vi "Live Report.vi"(8 "error in":errorcluster, 11 "TDMS in":refnum<class "TDMS.lvclass">) -> (0 "error out":errorcluster, 3 "TDMS out":refnum<class "TDMS.lvclass">)   [LabVIEW 2019, in "TDMS.lvlib" / "TDMS.lvclass"]
uses:
  TDMS.lvclass
  TDMS.lvclass/TDMS.ctl
  Report Viewer/Custom Controls/Browse Tools.ctl
  <vilib>/Utility/tdmsutil.llb/fileViewerConfigData.ctl
  Report Viewer/Report Viewer.lvclass
panel:
  out "TDMS File":string="Press 'Refresh Data' to load the latest data from the live report."
  in  "Display Format":T1(ring)
  in  "Refresh Data":bool
  in  "Save Data":bool
  in  "Settings":bool
  in  "Save Graph":bool
  in  "Finished":bool
  in  "File contents":string[](tree)=["\"\u0000\u0000\u0000\u0002\u0000\u0000\u0000+Halt Mode Running_11:25:18.755 AM 11/6/2019\u0000\u0000\u0000\nPJB1_S CH0\""]
  in  "Properties / Values / Graph":T2(tab)=enum."Analog values (graph)"
  in  "Properties":i32(listbox)
  in  "Raw data values":i32(listbox)=-1
  out "Waveform Graph":waveform(dbl)[](graph)=[{"t0"=timestamp(0 s since 1904-01-01), "dt"=1.0, "Y"=[]}]
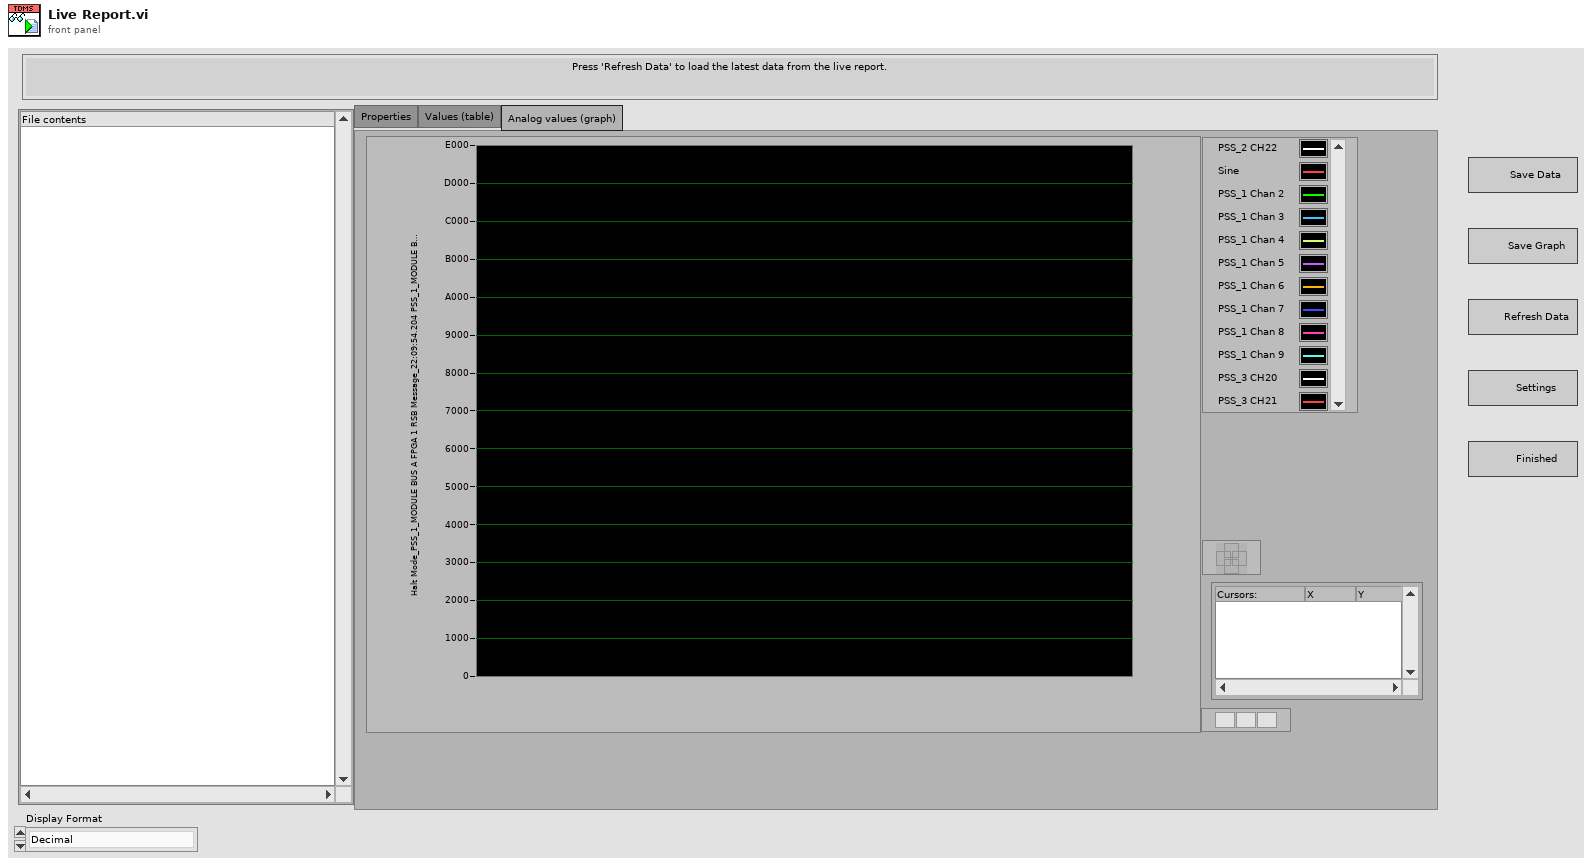
[diagram p1: front panel]
types:
  T1 = enum16{"Decimal", "Scientific", "Engineering", "Binary", "Octal", "Hexadecimal"}
  T2 = enum32{"Properties", "Values (table)", "Analog values (graph)"}
  T3 = typedef "fileViewerConfigData.ctl" = cluster{"Show all (table)":bool, "Show all (graph)":bool, "limit (table)":u64, "limit (graph)":u64, "no show":bool, "start (table)":u64, "start (graph)":u64}
  T4 = typedef "Report Viewer.lvlib/Report Viewer.lvclass/Browse Tools.ctl" = cluster{"Group":string, "Channel":string, "TDMS View Cfg":T3}
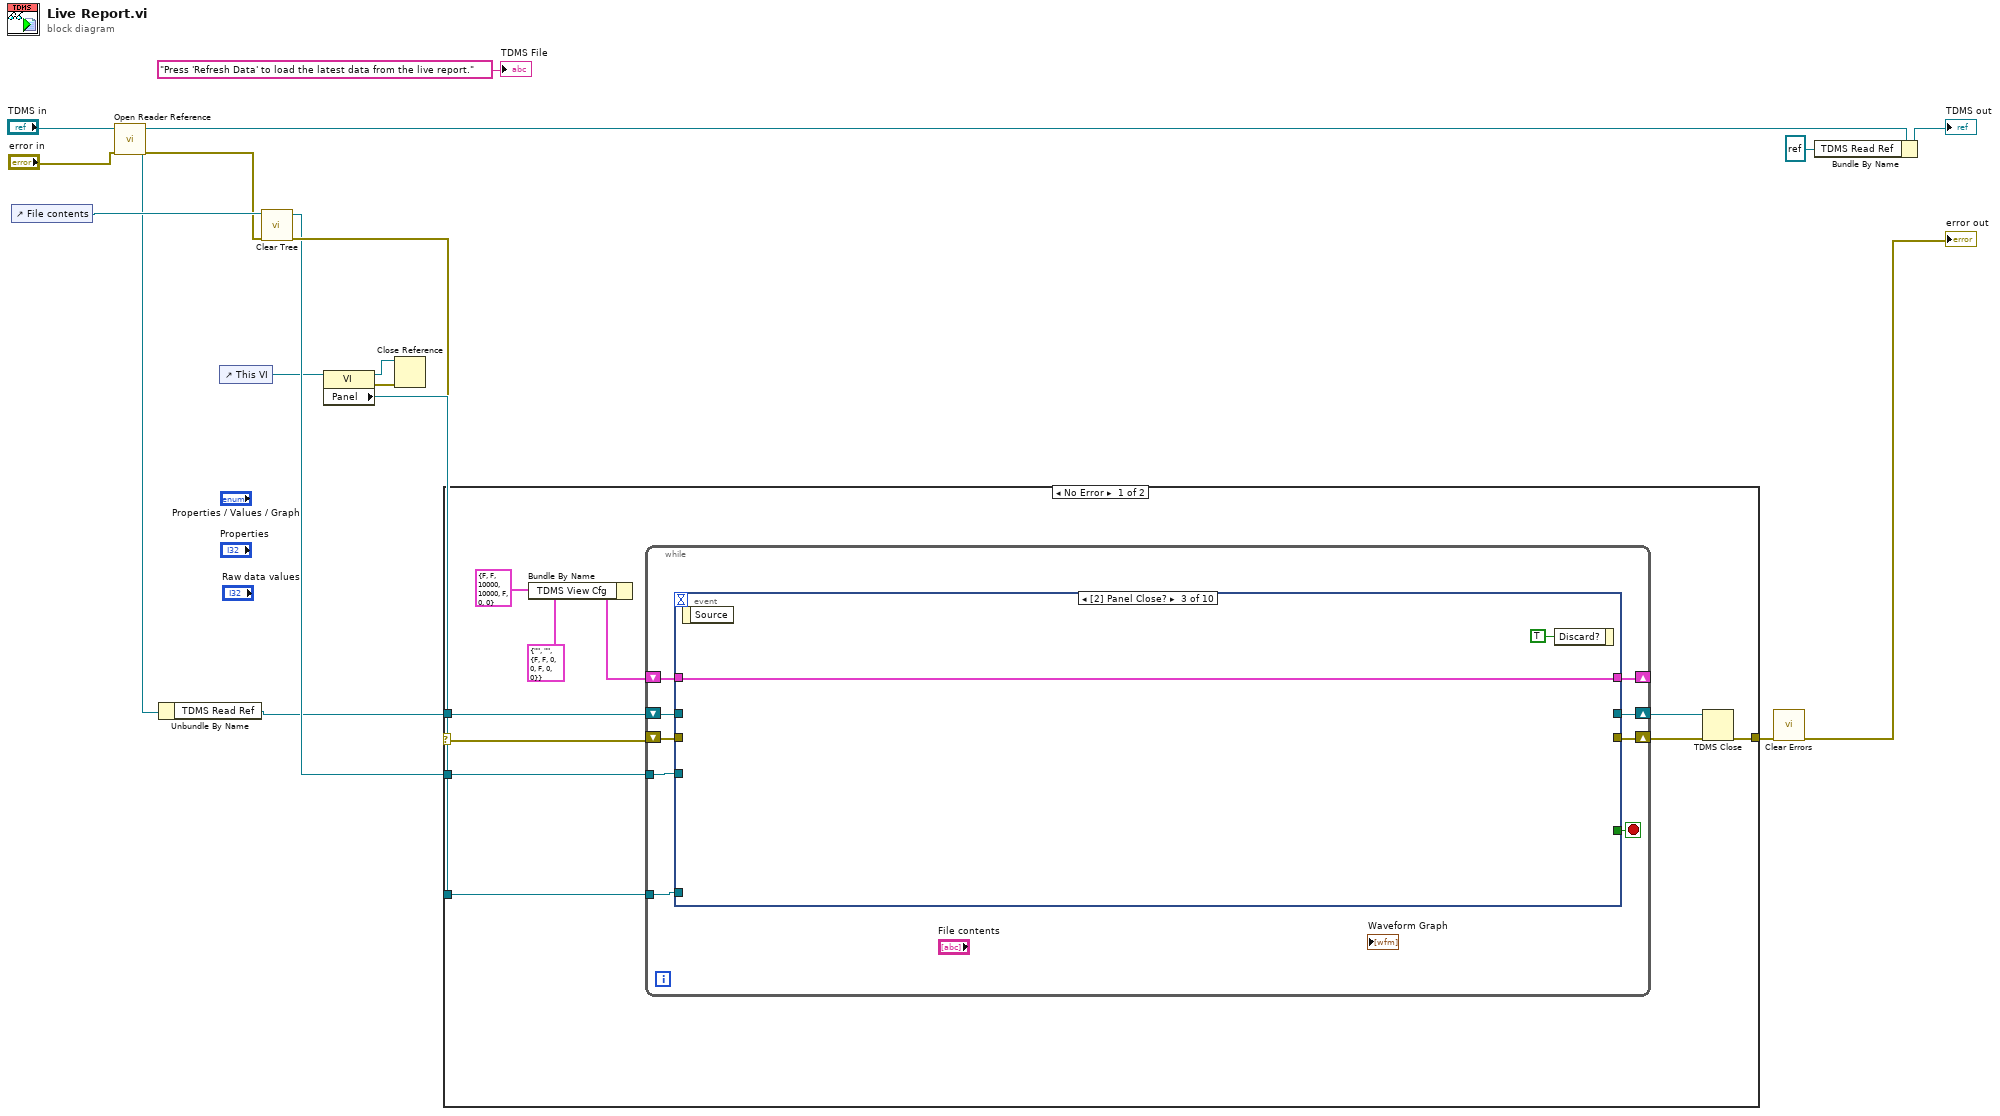
[diagram p0: block diagram]
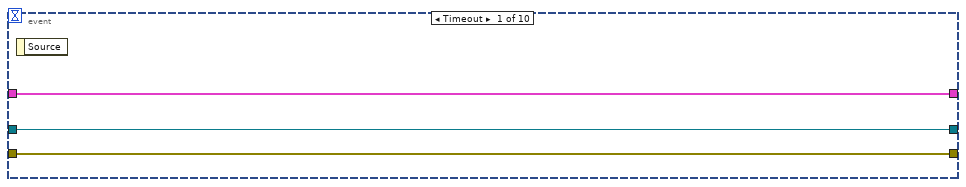
[diagram p2: hidden frame]
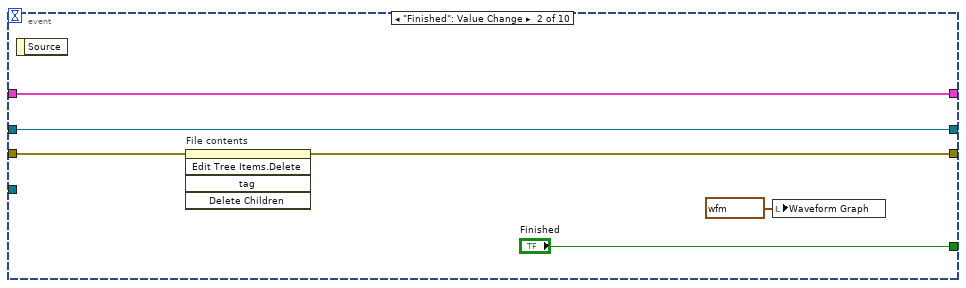
[diagram p3: hidden frame]
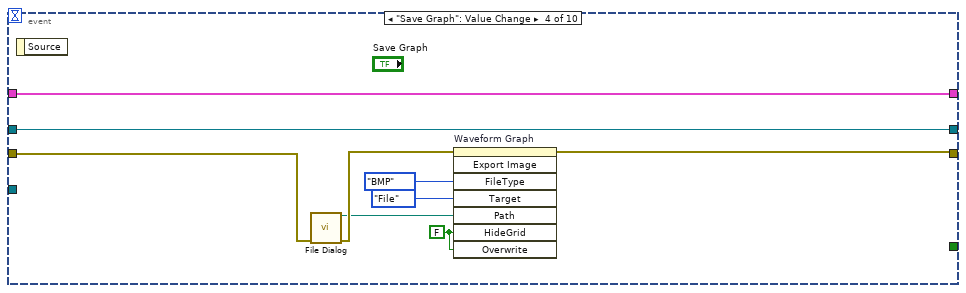
[diagram p4: hidden frame]
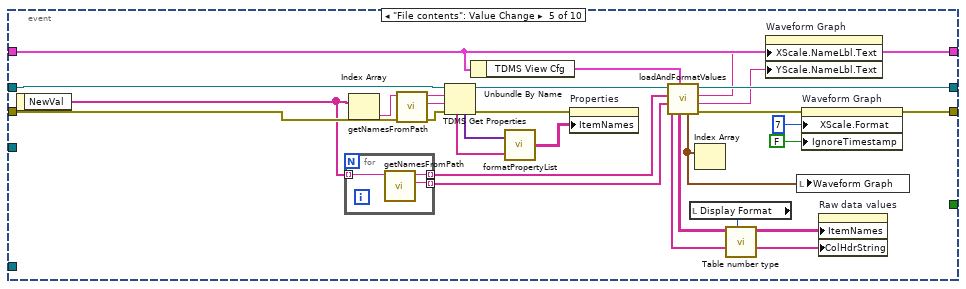
[diagram p5: hidden frame]
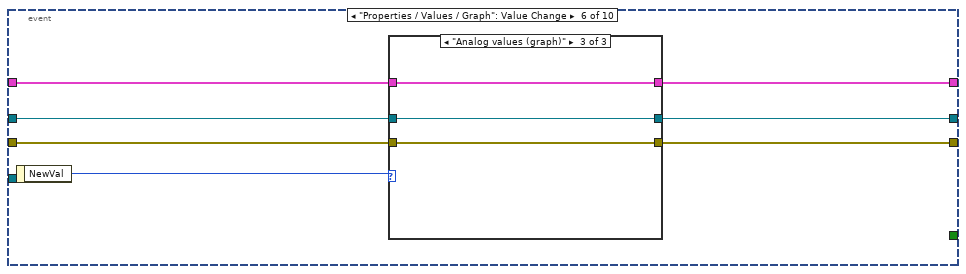
[diagram p6: hidden frame]
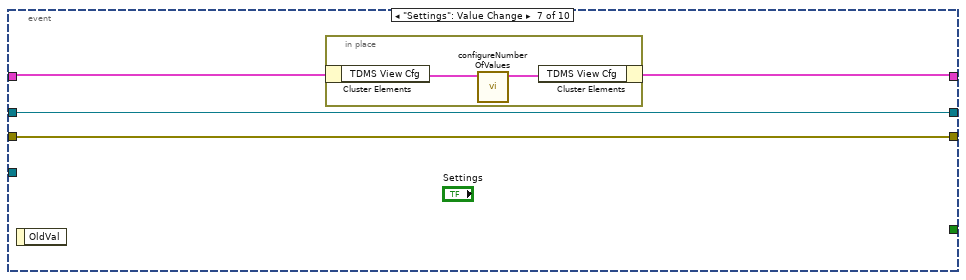
[diagram p9: hidden frame]
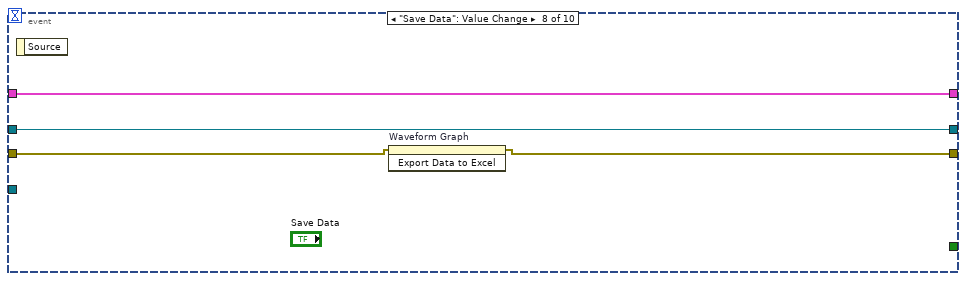
[diagram p10: hidden frame]
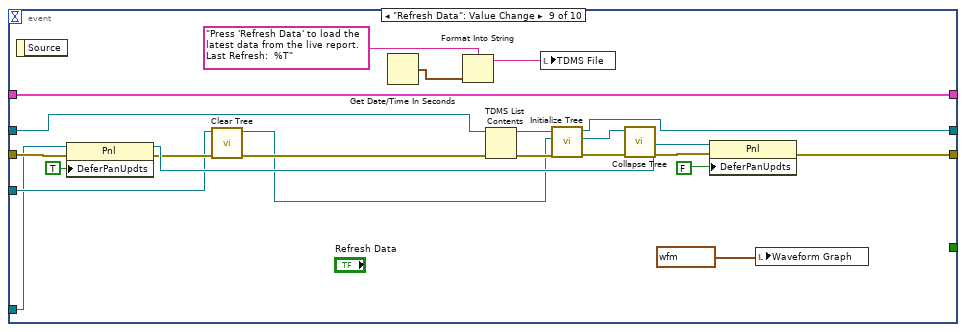
[diagram p11: hidden frame]
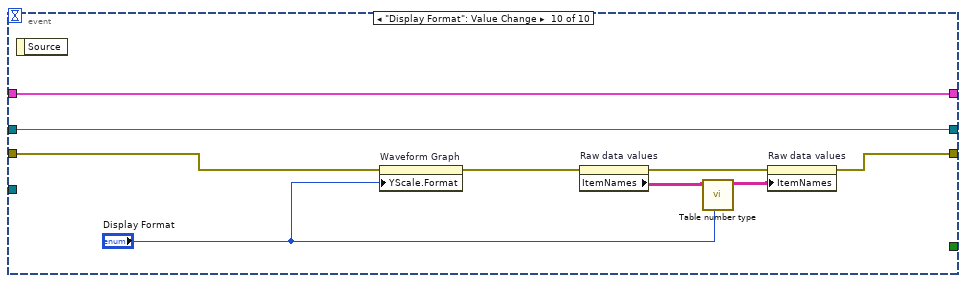
[diagram p12: hidden frame]
diagram:
  n1 = control-ref of="File contents"() -> (w16:refnum<vi>)
  n2 = call "Open Reader Reference.vi"("error in"="error in", "TDMS in"="TDMS in") -> ("error out"=w5:errorcluster, "TDMS out"=w4:refnum<class "TDMS.lvclass">)  [unwired: 8 in]
  n3 = Unbundle By Name(w4) -> ("TDMS Read Ref"=w6:refnum<k34>)
  n4 = control-ref of="This VI"() -> (w10:refnum<vi>)
  n5 = call "Clear Tree.vi"("error in"=w5, "reference"=w16) -> ("error out"=w14:errorcluster, "reference out"=w13:refnum<vi>)  [unwired: 8 in]
  n6 = property class="VI"(reference=w10) -> (reference out=w12:refnum<vi>, error out=w11:errorcluster, "Panel"=w15:refnum<vi>)  [unwired: 1 in]
  n7 = Close Reference(reference=w12, error in (no error)=w11) -> ()  [unwired: 1 out]
  n8 = case shown="No Error" w14 {
    selector: w14 -> [w20 w144]
    tunnel: [w27 w144] -> w9
    tunnel: w13 -> [w22 _]
    tunnel: w15 -> [w19 _]
    tunnel: w6 -> [w18 _]
    frame No Error {
      n9 = Bundle By Name(cluster=T4 {"Group"="", "Channel"="", "TDMS View Cfg"={"Show all (table)"=FALSE, "Show all (graph)"=FALSE, "limit (table)"=0, "limit (graph)"=0, "no show"=FALSE, "start (table)"=0, "start (graph)"=0}} ("Cluster"), "TDMS View Cfg"=T3 {"Show all (table)"=FALSE, "Show all (graph)"=FALSE, "limit (table)"=10000, "limit (graph)"=10000, "no show"=FALSE, "start (table)"=0, "start (graph)"=0} ("TDMS File Viewer Configuration")) -> (w24:T4)
      n10 = while {
        shift-right: [w34] -> w26
        shift-left: w20 -> [w35]
        shift-right: [w29] -> w21
        shift-left: w18 -> [w36]
        shift-right: [w31] -> _
        shift-left: w24 -> [w32]
        tunnel: w22 -> [w30]
        tunnel: w19 -> [w28]
        stop <- w33 stop-if-true
        n11 = event shown="[2] Panel Close?" {
          selector: _ -> [_ _ _ _ _ _ _ _ _ _]
          dyn-events: _ -> [_ _ _ _ _ _ _ _ _ _]
          timeout: _ -> [_ _ _ _ _ _ _ _ _ _]
          tunnel: w36 -> [w37 w42 _ w47 w61 w92 w103 w109 w118 w141]
          tunnel: w35 -> [w39 w40 _ w54 w83 w88 w104 w111 w124 w142]
          tunnel: [w39 w40 _ w53 w66 w87 w104 w110 w128 w139] -> w34
          tunnel: [_ "Finished" _ _ _ _ _ _ _ _] -> w33
          tunnel: w32 -> [w38 w43 w46 w55 w74 w91 w106 w112 w134 w143]
          tunnel: [w38 w43 w46 w55 w74 w90 w105 w112 w134 w143] -> w31
          tunnel: w30 -> [_ _ _ _ _ _ _ _ w121 _]
          tunnel: [w37 w42 _ w47 w62 w89 w103 w109 w127 w141] -> w29
          tunnel: w28 -> [_ _ _ _ _ _ _ _ w120 _]
          event Timeout {
            n12 = event-data() -> ()  [unwired: 1 in, 1 out]
          }
          event "Finished": Value Change {
            n13 = event-data() -> ()  [unwired: 1 in, 1 out]
            n14 = invoke on="File contents" class="Tree (strict)" method="Edit Tree Items.Delete"(error in=w40) -> ()  [unwired: 4 in, 5 out]
            n15 = local write "Waveform Graph"(waveform(dbl)[] [{"t0"=timestamp(0 s since 1904-01-01), "dt"=1.0, "Y"=[]}] ("Waveform Graph")) -> ()
          }
          event Panel Close? {
            n16 = event-data() -> ()  [unwired: 1 in, 1 out]
            n17 = event-data("Discard?"=TRUE) -> ()  [unwired: 1 in, 1 out]
          }
          event "Save Graph": Value Change {
            w48 = FALSE ("Hide Grid")
            n18 = event-data() -> ()  [unwired: 1 in, 1 out]
            n19 = call "File Dialog"("error in"=w54) -> ("selected path"=w49:path, "error out"=w52:errorcluster)  [unwired: 11 in, 2 out]
            n20 = invoke on="Waveform Graph" class="WFGraph (strict)" method="Export Image"(error in=w52, "FileType"=enum32{"BMP", "EPS", "EMF", "PICT"}."BMP" ("File Type"), "Target"=enum32{"File", "Clipboard"}."File", "Path"=w49, "HideGrid"=w48, "Overwrite"=w48) -> (error out=w53:errorcluster)  [unwired: 2 in, 7 out]
          }
          event "File contents": Value Change {
            n21 = event-data() -> ("NewVal"=w71:string[])  [unwired: 1 in]
            n22 = for {
              tunnel: w71 -> [w86] mode=indexing
              tunnel: [w85] -> w70 mode=indexing
              tunnel: [w84] -> w69 mode=indexing
              n23 = call <vilib>:"getNamesFromPath.vi"("tree path"=w86) -> ("channel"=w84:string, "group"=w85:string)  [unwired: 1 in, 4 out]
            }
            n24 = Index Array(array=w71) -> (element=w75:string)  [unwired: 1 in]
            n25 = call <vilib>:"getNamesFromPath.vi"("error in (no error)"=w83, "tree path"=w75) -> ("error out"=w82:errorcluster, "channel"=w80:string, "group"=w81:string)  [unwired: 3 out]
            n26 = TDMS Get Properties(8:w82, 9:w80, 10:w81, 11:w61) -> (0:w76:errorcluster, 3:w72:refnum<k34>, 4:w79:variant[], 6:w78:string[])  [unwired: 4 out]
            n27 = Unbundle By Name(w74) -> ("TDMS View Cfg"=w73:T3)
            n28 = call <vilib>:"formatPropertyList.vi"("property names"=w78, "property values"=w79) -> ("strings"=w77:string[][])
            n29 = property on="Properties" class="MCListbox (strict)"(error in=w76, "ItemNames"=w77) -> ()  [unwired: 1 in, 2 out]
            n30 = call <vilib>:"loadAndFormatValues.vi"("configuration"=w73, "channel names"=w69, "group names"=w70, "tdms file"=w72) -> ("error out"=w67:errorcluster, "graph y names"=w59:string, "graph x names"=w60:string, "tdms file out"=w62:refnum<k34>, "waveform values"=w63:waveform(dbl)[], "table values"=w57:string[][], "table headers"=w68:string[])  [unwired: 1 in]
            n31 = local read "Display Format"() -> (w56:T1)
            n32 = Index Array(array=w63) -> ()  [unwired: 1 in, 1 out]
            n33 = call "Table number type.vi"("Y Scale.Display Format:Format"=w56, "Item Names in"=w57) -> ("Item Names out"=w58:string[][])  [unwired: 9 in]
            n34 = property on="Waveform Graph" class="WFGraph (strict)"("XScale.NameLbl.Text"=w60, "YScale.NameLbl.Text"=w59) -> ()  [unwired: 2 in, 2 out]
            n35 = local write "Waveform Graph"(w63) -> ()
            n36 = property on="Waveform Graph" class="WFGraph (strict)"(error in=w67, "XScale.Format"=u8 7 ("X Scale.Display Format:Format"), "IgnoreTimestamp"=FALSE ("Ignore Timestamp")) -> (error out=w66:errorcluster)  [unwired: 1 in, 1 out]
            n37 = property on="Raw data values" class="MCListbox (strict)"("ItemNames"=w58, "ColHdrString"=w68) -> ()  [unwired: 2 in, 2 out]
          }
          event "Properties / Values / Graph": Value Change {
            n38 = event-data() -> ("NewVal"=w93:T2)  [unwired: 1 in]
            n39 = case shown="\"Analog values (graph)\"" w93 {
              tunnel: w92 -> [w96 w98 w101]
              tunnel: [w96 w98 w101] -> w89
              tunnel: w91 -> [w95 w99 w102]
              tunnel: [w95 w99 w102] -> w90
              tunnel: w88 -> [w94 w97 w100]
              tunnel: [w94 w97 w100] -> w87
              frame "Properties", Default {
              }
              frame "Values (table)" {
              }
              frame "Analog values (graph)" {
              }
            }
          }
          event "Settings": Value Change {
            n40 = event-data() -> ()  [unwired: 1 in, 1 out]
            n41 = in-place {
              n42 = in-place-cluster #1(w106) -> ("TDMS View Cfg"=w108:T3)
              n43 = call <vilib>:"configureNumberOfValues.vi"("TDMS File Viewer Configuration"=w108) -> ("TDMS File Viewer Configuration Out"=w107:T3)  [unwired: 10 out]
              n44 = in-place-cluster #1("TDMS View Cfg"=w107) -> (w105:T4)
            }
          }
          event "Save Data": Value Change {
            n45 = event-data() -> ()  [unwired: 1 in, 1 out]
            n46 = invoke on="Waveform Graph" class="WFGraph (strict)" method="Export Data to Excel"(error in=w111) -> (error out=w110:errorcluster)  [unwired: 2 in, 2 out]
          }
          event "Refresh Data": Value Change {
            n47 = event-data() -> ()  [unwired: 1 in, 1 out]
            n48 = property class="Pnl"(reference=w120, error in=w124, "DeferPanUpdts"=TRUE ("Defer Panel Updates")) -> (reference out=w123:refnum<vi>, error out=w122:errorcluster)
            n49 = call "Clear Tree.vi"("error in"=w122, "reference"=w121) -> ("error out"=w119:errorcluster, "reference out"=w113:refnum<vi>)  [unwired: 8 in]
            n50 = Get Date/Time In Seconds() -> (seconds since 1Jan1904=w115:timestamp)
            n51 = Format Into String(format string="Press 'Refresh Data' to load the latest data from the live report. Last Refresh:  %T" ("TDMS File"), w115) -> (resulting string=w114:string)  [unwired: 2 in, 1 out]
            n52 = TDMS List Contents(4:w119, 7:w118) -> (0:w117:errorcluster, 3:w129:refnum<k34>)  [unwired: 1 in, 2 out]
            n53 = local write "TDMS File"(w114) -> ()
            n54 = call "Initialize Tree.vi"("error in"=w117, "reference"=w113, "tdms file"=w129) -> ("error out"=w131:errorcluster, "tree reference out"=w132:refnum<vi>, "tdms file out"=w127:refnum<k34>)  [unwired: 6 in]
            n55 = call "Collapse Tree.vi"("error in (no error)"=w131, "Tree Ref in"=w132) -> ("error out"=w130:errorcluster)  [unwired: 8 in, 1 out]
            n56 = property class="Pnl"(reference=w123, error in=w130, "DeferPanUpdts"=FALSE ("Defer Panel Updates")) -> (error out=w128:errorcluster)  [unwired: 1 out]
            n57 = local write "Waveform Graph"(waveform(dbl)[] [{"t0"=timestamp(0 s since 1904-01-01), "dt"=1.0, "Y"=[]}] ("Waveform Graph")) -> ()
          }
          event "Display Format": Value Change {
            n58 = event-data() -> ()  [unwired: 1 in, 1 out]
            n59 = property on="Waveform Graph" class="WFGraph (strict)"(error in=w142, "YScale.Format"="Display Format") -> (error out=w140:errorcluster)  [unwired: 1 in, 1 out]
            n60 = property on="Raw data values" class="MCListbox (strict)"(error in=w140) -> (error out=w138:errorcluster, "ItemNames"=w137:string[][])  [unwired: 1 in, 1 out]
            n61 = call "Table number type.vi"("Y Scale.Display Format:Format"="Display Format", "Item Names in"=w137) -> ("Item Names out"=w136:string[][])  [unwired: 9 in]
            n62 = property on="Raw data values" class="MCListbox (strict)"(error in=w138, "ItemNames"=w136) -> (error out=w139:errorcluster)  [unwired: 1 in, 1 out]
          }
        }
      }
      n63 = TDMS Close(8:w26, 11:w21) -> (0:w27:errorcluster)  [unwired: 1 out]
    }
    frame Error {
    }
  }
  n64 = call <vilib>:"Clear Errors.vi"("error in (no error)"=w9) -> ("error out"=→"error out":errorcluster)  [unwired: 5 in, 1 out]
  n65 = Bundle By Name(cluster=w4, "TDMS Read Ref"=refnum<k34> refnum) -> (→"TDMS out":refnum<class "TDMS.lvclass">)
  "TDMS File" <- "Press 'Refresh Data' to load the latest data from the live report." ("TDMS File")
